vi "PicoScopeospaOpen.vi"(5 "Serial Number":string, 7 "Use Serial Number":bool, 8 "error in (no error)":errorcluster, 9 "Mode":u16(ring) items=["Dialog On Error", "no dialog - CloseUnit and Stop", "no dialog - Continue", "no dialog - Stop"], 10 "Resolution":u32(ring) items=["8-bit"=0, "12-bit"=1, "14-bit"=2, "15-bit"=3, "16-bit"=4, "10-bit"=10]) -> (0 "error out":errorcluster, 1 "Max ADC value":i16, 2 "Device Info":T1, 3 "handle out":i16, 4 "psospa Units":string, 6 "serialLth":i16)   [LabVIEW 2024]
doc: "This VI manages listing and opens devices with device details."
uses:
  psospa.dll
panel:
  out "minValue":i16
  # "NO 32-bit support for psospa.dll\n\n64-bit LabVIEW ONLY"
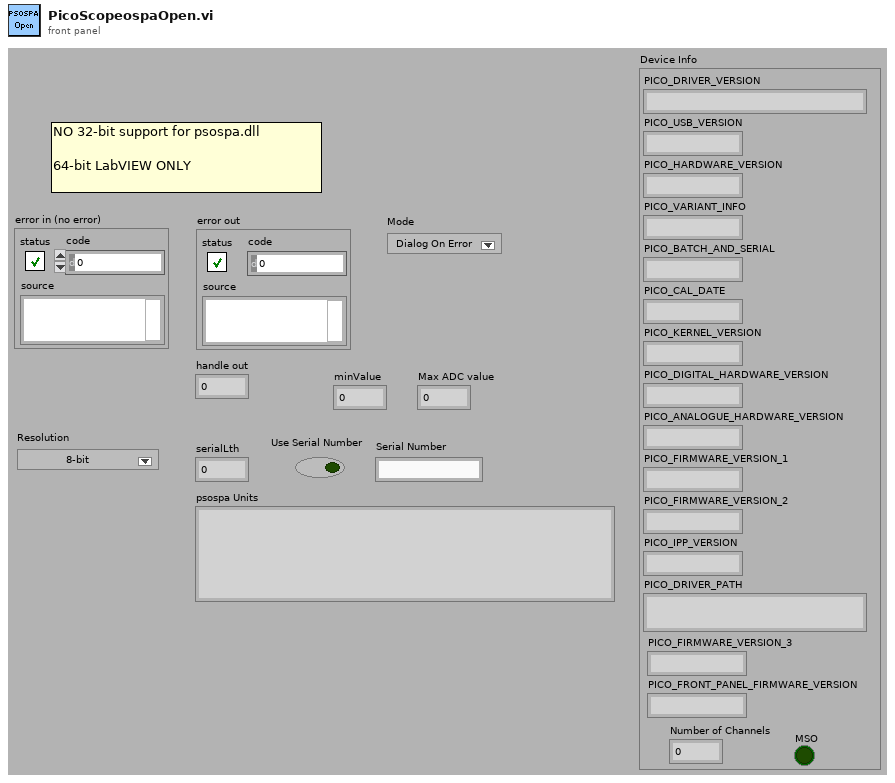
[diagram p1: front panel]
types:
  T1 = cluster{"PICO_DRIVER_VERSION":string, "PICO_USB_VERSION":string, "PICO_HARDWARE_VERSION":string, "PICO_VARIANT_INFO":string, "PICO_BATCH_AND_SERIAL":string, "PICO_CAL_DATE":string, "PICO_KERNEL_VERSION":string, "PICO_DIGITAL_HARDWARE_VERSION":string, "PICO_ANALOGUE_HARDWARE_VERSION":string, "PICO_FIRMWARE_VERSION_1":string, "PICO_FIRMWARE_VERSION_2":string, "PICO_IPP_VERSION":string, "PICO_DRIVER_PATH":string, "PICO_FIRMWARE_VERSION_3":string, "PICO_FRONT_PANEL_FIRMWARE_VERSION":string, "Number of Channels":i16, "MSO":bool}
  T2 = cluster{"status":bool, "code":u32, "source":string}
  T3 = cluster{"PICO_DRIVER_VERSION":string, "PICO_USB_VERSION":string, "PICO_HARDWARE_VERSION":string, "PICO_VARIANT_INFO":string, "PICO_BATCH_AND_SERIAL":string, "PICO_CAL_DATE":string, "PICO_KERNEL_VERSION":string, "PICO_DIGITAL_HARDWARE_VERSION":string, "PICO_ANALOGUE_HARDWARE_VERSION":string, "PICO_FIRMWARE_VERSION_1":string, "PICO_FIRMWARE_VERSION_2":string, "PICO_IPP_VERSION":string, "PICO_DRIVER_PATH":string, "PICO_FIRMWARE_VERSION_3":string, "PICO_FRONT_PANEL_FIRMWARE_VERSION":string}
  T4 = cluster{"PICO_DRIVER_VERSION":string, "PICO_USB_VERSION":string, "PICO_HARDWARE_VERSION":string, "PICO_VARIANT_INFO":string, "PICO_BATCH_AND_SERIAL":string, "PICO_CAL_DATE":string, "PICO_KERNEL_VERSION":string, "PICO_DIGITAL_HARDWARE_VERSION":string, "PICO_ANALOGUE_HARDWARE_VERSION":string, "PICO_FIRMWARE_VERSION_1":string, "PICO_FIRMWARE_VERSION_2":string, "PICO_IPP_VERSION":string, "PICO_DRIVER_PATH":string, "PICO_FIRMWARE_VERSION_3":string, "PICO_FRONT_PANEL_FIRMWARE_VERSION":string, i16, bool}
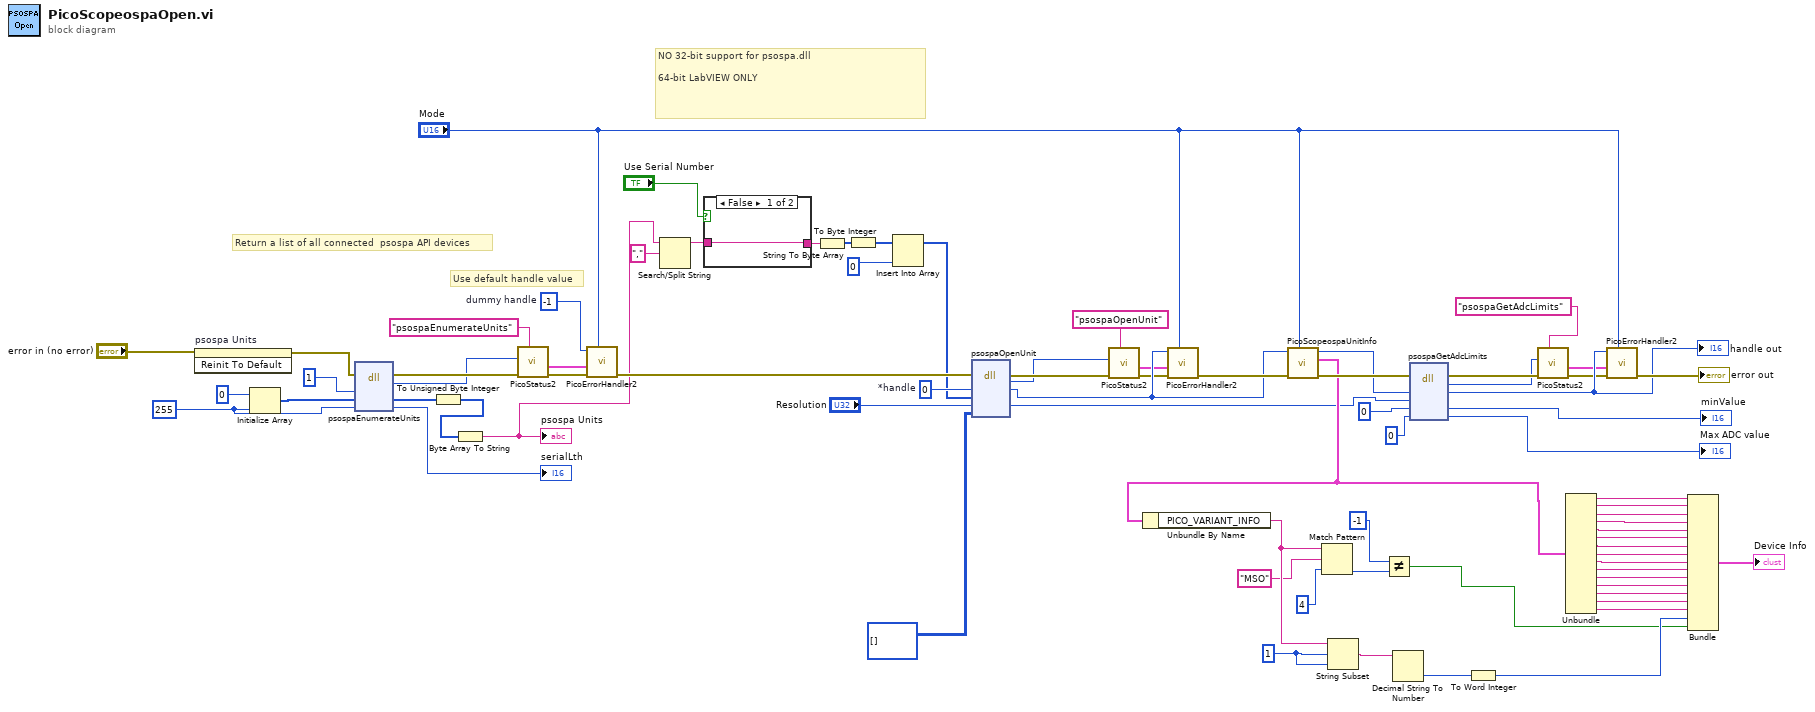
[diagram p0: block diagram]
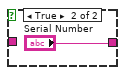
[diagram p2: hidden frame]
diagram:
  w29 = i16 -1  # dummy handle
  w33 = i16 255 ("dimension size")
  w67 = 1 ("offset (0)")
  w41 = i16 0  # *handle
  # "NO 32-bit support for psospa.dll\n\n64-bit LabVIEW ONLY"
  # "Use default handle value"
  # "Return a list of all connected  psospa API devices"
  n1 = invoke on="psospa Units" class="Str" method="Reinit To Default"(error in="error in (no error)") -> (error out=w30:errorcluster)  [unwired: 2 in, 2 out]
  n2 = Initialize Array(i8 0 ("U8"), w33) -> (w35:i8[])
  n3 = dll-call lib="F:/Picoscope3000e/Scope_LabView/ps3000e/Treiber_und_SubVis/psospa.dll" fn="psospaEnumerateUnits"(error in=w30, "count"=i16 1, "serials"=w35, "serialLth"=w33) -> (error out=w24:errorcluster, "PICO_STATUS"=w23:u32, "serials"=w31:i8[], "serialLth"=→"serialLth":i16)  [unwired: 3 in, 1 out]
  n4 = To Unsigned Byte Integer(number=w31) -> (unsigned 8bit integer=w32:u8[])
  n5 = Byte Array To String(unsigned byte array=w32) -> (string=w14:string)
  "psospa Units" <- w14
  n6 = call "PicoStatus2.vi"("PICO source"="psospaEnumerateUnits" ("source"), "Error in"=w24, "PICO STATUS"=w23) -> ("error out"=w22:errorcluster, "PICO_STATUS out"=w21:T2)  [unwired: 5 in]
  n7 = call "PicoErrorHandler2.vi"("Mode"="Mode", "error in (no error)"=w22, "PICO_STATUS in"=w21, "handle In"=w29) -> ("error out"=w40:errorcluster)  [unwired: 7 in]
  n8 = Search/Split String(string=w14, search string/char (-)=",") -> (substring before match=w19:string)  [unwired: 1 in, 2 out]
  n9 = case shown="False" "Use Serial Number" {
    tunnel: w19 -> [w78 _]
    tunnel: [w78 "Serial Number"] -> w15
    frame False {
    }
    frame True {
    }
  }
  n10 = String To Byte Array(string=w15) -> (unsigned byte array=w17:u8[])
  n11 = To Byte Integer(number=w17) -> (8bit integer=w18:i8[])
  n12 = Insert Into Array(array=w18, new element=i8 0 ("new element/subarray")) -> (w12:i8[])  [unwired: 1 in]
  n13 = dll-call lib="F:/Picoscope3000e/Scope_LabView/ps3000e/Treiber_und_SubVis/psospa.dll" fn="psospaOpenUnit" ("ps3000.dll:_ps3000_open_unit@0")(error in=w40, "handle"=w41, "serial"=w12, "resolution"="Resolution", "powerDetails"=u8[][] []) -> (error out=w8:errorcluster, "PICO_STATUS"=w7:u32, "handle"=w28:i16, "resolution"=w38:u32)  [unwired: 4 in, 1 out]
  n14 = call "PicoStatus2.vi"("PICO source"="psospaOpenUnit" ("source"), "Error in"=w8, "PICO STATUS"=w7) -> ("error out"=w11:errorcluster, "PICO_STATUS out"=w10:T2)  [unwired: 5 in]
  n15 = call "PicoErrorHandler2.vi"("Mode"="Mode", "error in (no error)"=w11, "PICO_STATUS in"=w10, "handle In"=w28) -> ("error out"=w77:errorcluster)  [unwired: 7 in]
  n16 = call "PicoScopeospaUnitInfo.vi"("Mode"="Mode", "error in (no error)"=w77, "handle in"=w28) -> ("error out"=w60:errorcluster, "Unit Info"=w53:T3, "handle out"=w58:i16)  [unwired: 6 in]
  n17 = Unbundle By Name(w53) -> ("PICO_VARIANT_INFO"=w66:string)
  n18 = Match Pattern(string=w66, regular expression="MSO", offset (0)=4) -> (offset past match=w63:i32)  [unwired: 3 out]
  n19 = String Subset(string=w66, offset (0)=w67, length (rest)=w67) -> (substring=w46:string)
  n20 = Not Equal?(x=-1, y=w63) -> (x != y?=w27:bool)
  n21 = Decimal String To Number(string=w46) -> (number=w43:i32)  [unwired: 2 in, 1 out]
  n22 = dll-call lib="F:/Picoscope3000e/Scope_LabView/ps3000e/Treiber_und_SubVis/psospa.dll" fn="psospaGetAdcLimits" ("ps3000.dll:_ps3000_open_unit@0")(error in=w60, "handle"=w58, "resolution"=w38, "minValue"=i16 0, "maxValue"=i16 0 ("manValue")) -> (error out=w3:errorcluster, "PICO_STATUS"=w2:u32, "handle"=w59:i16, "minValue"=→"minValue":i16, "maxValue"=→"Max ADC value":i16)  [unwired: 3 in, 1 out]
  "handle out" <- w59
  n23 = To Word Integer(number=w43) -> (16bit integer=w42:i16)
  n24 = call "PicoStatus2.vi"("PICO source"="psospaGetAdcLimits" ("source"), "Error in"=w3, "PICO STATUS"=w2) -> ("error out"=w6:errorcluster, "PICO_STATUS out"=w5:T2)  [unwired: 5 in]
  n25 = Unbundle(w53) -> ("PICO_DRIVER_VERSION"=w76:string, "PICO_USB_VERSION"=w75:string, "PICO_HARDWARE_VERSION"=w74:string, "PICO_VARIANT_INFO"=w73:string, "PICO_BATCH_AND_SERIAL"=w72:string, "PICO_CAL_DATE"=w71:string, "PICO_KERNEL_VERSION"=w70:string, "PICO_DIGITAL_HARDWARE_VERSION"=w69:string, "PICO_ANALOGUE_HARDWARE_VERSION"=w68:string, "PICO_FIRMWARE_VERSION_1"=w52:string, "PICO_FIRMWARE_VERSION_2"=w51:string, "PICO_IPP_VERSION"=w50:string, "PICO_DRIVER_PATH"=w49:string, "PICO_FIRMWARE_VERSION_3"=w48:string, "PICO_FRONT_PANEL_FIRMWARE_VERSION"=w47:string)
  n26 = call "PicoErrorHandler2.vi"("Mode"="Mode", "error in (no error)"=w6, "PICO_STATUS in"=w5, "handle In"=w59) -> ("error out"=→"error out":errorcluster)  [unwired: 7 in]
  n27 = Bundle("PICO_DRIVER_VERSION"=w76, "PICO_USB_VERSION"=w75, "PICO_HARDWARE_VERSION"=w74, "PICO_VARIANT_INFO"=w73, "PICO_BATCH_AND_SERIAL"=w72, "PICO_CAL_DATE"=w71, "PICO_KERNEL_VERSION"=w70, "PICO_DIGITAL_HARDWARE_VERSION"=w69, "PICO_ANALOGUE_HARDWARE_VERSION"=w68, "PICO_FIRMWARE_VERSION_1"=w52, "PICO_FIRMWARE_VERSION_2"=w51, "PICO_IPP_VERSION"=w50, "PICO_DRIVER_PATH"=w49, "PICO_FIRMWARE_VERSION_3"=w48, "PICO_FRONT_PANEL_FIRMWARE_VERSION"=w47, w42, w27) -> (→"Device Info":T4)  [unwired: 1 in]
